vi "vission comm test.vi"() -> ()   [LabVIEW 2009]
uses:
  behaviors/driveable path/drivable paths global.vi
  <vilib>/rvi/DataTransferAndStorage/Container/XNode/niFpgaContainer.xnode
  <vilib>/rvi/FIFO/Fifo_Resource/nirvififoUniquifyingName.vi
panel:
  in  "Invert Polarity?":bool
  out "driveable path lengths (lines)":u16[](array[numeric])
  out "line  raw serial port data":i16
  out "Number of Elements to Read":u32
  in  "baud rate (9600)":u32=9600
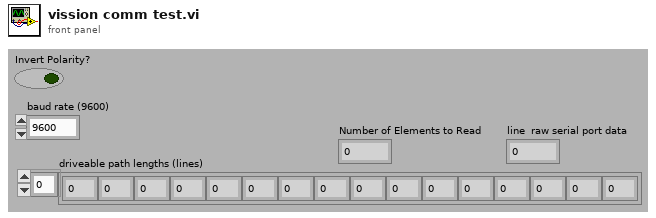
[diagram p1: front panel]
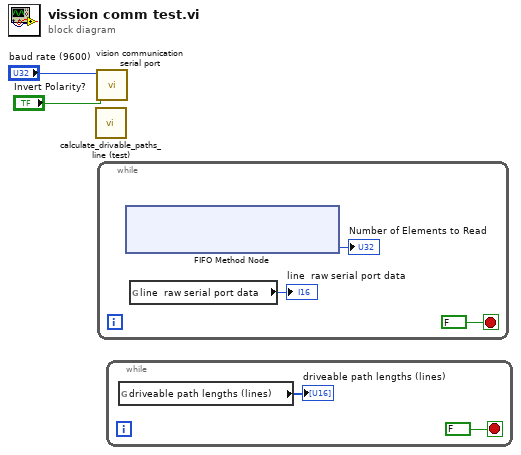
[diagram p0: block diagram]
diagram:
  n1 = call "calculate_drivable_paths_line (test).vi"() -> ()  [unwired: 1 in]
  n2 = call "vision communication serial port.vi"("Invert Polarity?"="Invert Polarity?", "baud rate (9600)"="baud rate (9600)") -> ()  [unwired: 10 in]
  n3 = while {
    stop <- FALSE stop-if-true
    n4 = xnode ("FIFO Method Node")() -> ("Number of Elements to Read"=→"Number of Elements to Read":u32)  [unwired: 1 in, 1 out]
    n5 = global read "drivable paths global.vi" "line  raw serial port data"() -> (→"line  raw serial port data":i16)
  }
  n6 = while {
    stop <- FALSE stop-if-true
    n7 = global read "drivable paths global.vi" "driveable path lengths (lines)"() -> (→"driveable path lengths (lines)":u16[])
  }
